vi "CRYSet table cell size.vi"(10 "Colum size":i32, 11 "Table":refnum<vi>) -> ()   [LabVIEW 2013]
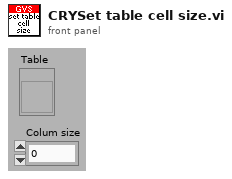
[diagram p1: front panel]
types:
  T1 = typedef "LVBoundsTypeDef.ctl" = cluster{"Width":u32, "Height":u32}
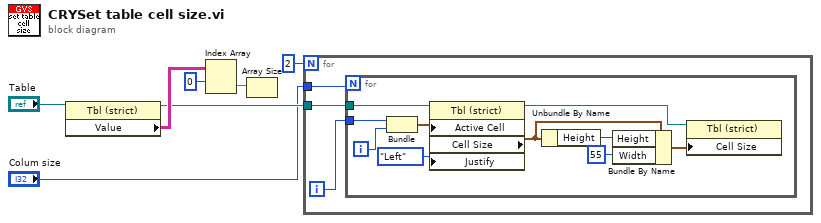
[diagram p0: block diagram]
diagram:
  n1 = property class="Tbl (strict)"(reference="Table") -> (reference out=w4:refnum<vi>, "Value"=w5:string[][])  [unwired: 1 in, 1 out]
  n2 = Index Array(array=w5, index (row)=0) -> (element=w6:string[])  [unwired: 1 in]
  n3 = Array Size(array=w6) -> ()  [unwired: 1 out]
  n4 = for {
    N: 2 -> [_]
    tunnel: "Colum size" -> [w10]
    tunnel: w4 -> [w9]
    i -> [w8]
    n5 = for {
      N: w10 -> [_]
      tunnel: w9 -> [w18]
      tunnel: w8 -> [w12]
      i -> [w20]
      n6 = Bundle(w12, w20) -> (w17:cluster{i32, i32})  [unwired: 1 out]
      n7 = property class="Tbl (strict)"(reference=w18, "Active Cell"=w17, "Justify"=enum16{"Left", "Center", "Right"}."Left" ("Active Cell:Cell Justification")) -> (reference out=w15:refnum<vi>, "Cell Size"=w16:T1)  [unwired: 1 in, 1 out]
      n8 = Unbundle By Name(w16) -> ("Height"=w19:u32)
      n9 = Bundle By Name(cluster=w16, "Height"=w19, "Width"=u32 55) -> (w14:T1)
      n10 = property class="Tbl (strict)"(reference=w15, "Cell Size"=w14) -> ()  [unwired: 1 in, 2 out]
    }
  }
